vi "test validation.vi"() -> ()   [LabVIEW 2013, in "TBM Tests.lvlib"]
uses:
  TBM Tests.lvlib
  root configuration/TBM configuration.lvclass
panel:
  out "no error":errorcluster
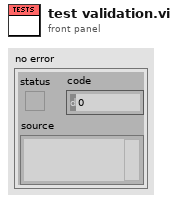
[diagram p1: front panel]
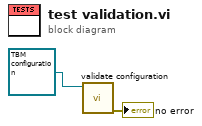
[diagram p0: block diagram]
diagram:
  n1 = call-dynamic "validate configuration.vi"("configuration in"=refnum<class "TBM configuration.lvclass"> refnum ("configuration")) -> ("error out"=→"no error":errorcluster)  [unwired: 9 in, 1 out]
